vi "Main.vi"() -> ()   [LabVIEW 2019]
doc: "This Continuous Measurement sample project is based on the Queued Message Handler template.\n\nThe Event Handling Loop generates messages based on user interface actions.\n\nThe Message Handling Loop processes messages generated by the Event Handling Loop, or by other messages. There are also Acquisition and Logging message handling loop subVIs, and a chart updating loop."
uses:
  <vilib>/Math Plots/2D Math Plots/2D Compass/2D Compass XCtrl/2D Compass.xctl
  Settings/Settings.ctl
  Acquisition/Hardware Configuration.ctl
  Logging/Logging Configuration.ctl
  controls/UI Data.ctl
  controls/UI Actions.ctl
  controls/UI Info Session.ctl
  Data Analysis/EstimateCluster.ctl
  controls/UI Display.ctl
  controls/Components State.ctl
  controls/State Type.ctl
  controls/Component Type.ctl
  Settings/Session Info.ctl
  controls/UI State.ctl
  support/Message Queue/Enqueue Message (Single).vi
  <vilib>/Utility/xml.llb/Write to XML File(string).vi
  <vilib>/Utility/error.llb/Error Cluster From Error Code.vi
  <vilib>/Utility/xml.llb/Read From XML File(string).vi
  <vilib>/Math Plots/2D Math Plots/2D Plot/2D Plot Datatype/2D Plot Datatype.lvclass
  <vilib>/ErrorRing/Error Ring.xnode
  Acquisition/Acquisition.lvlib
  Settings/Settings.lvlib
  Logging/Logging.lvlib
  support/User Event - Stop/User Event - Stop.lvlib
  support/Message Queue/Message Queue.lvlib
panel:
  out "Etat":string caption="Faux-Taon : Puissance-mètre"
  in  "Note":string
  out "Info sur la session":T1 {"Durée" format="%^<%H:%M:%S>T"}
  in  "Simuler":bool
  in  "Stop":bool
  in  "Start":bool
  in  "Calibrer":bool
  in  "Réinitialiser":bool
  in  "Charger session":bool
  in  "Enregistrer session":bool
  in  "Configuration":T2
  out "Longueur d'onde":dbl
  out "Puissance mesurée":dbl format="%#_3g"
  out "Position instantanée du faisceau vue de face":refnum<class "2D Plot Datatype.lvclass">[](xcontrol) caption="Position instantanée du faisceau"
  out "Graphique des mesures du laser":waveform(dbl)(graph)
  out "Status":string
  in  "Exit":bool
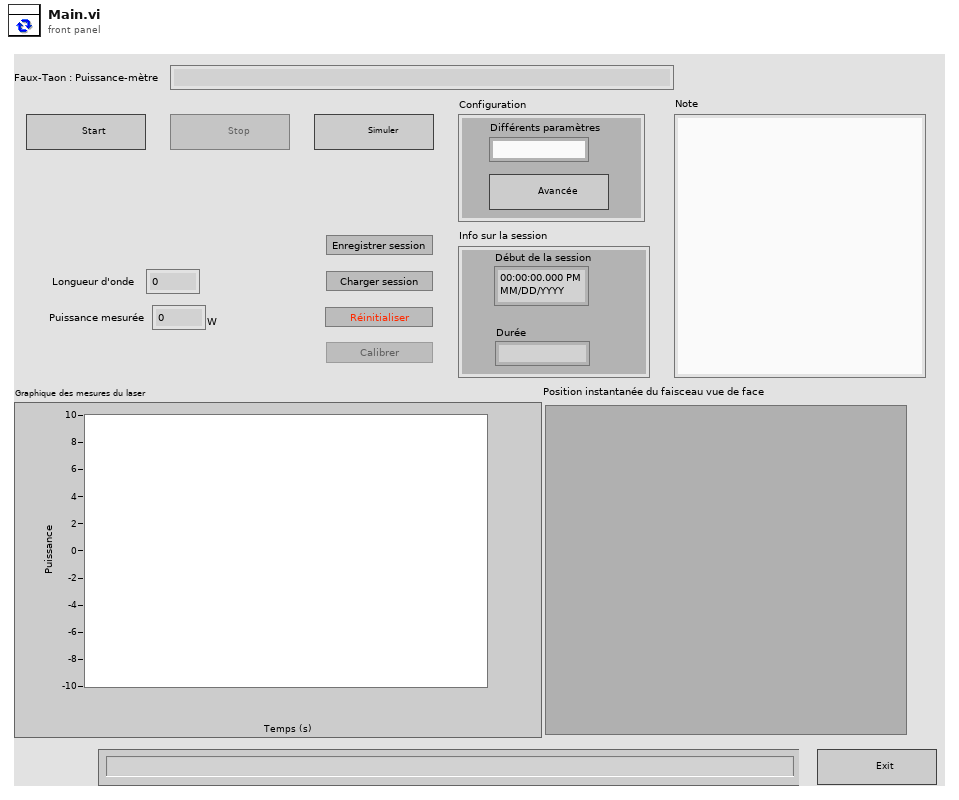
[diagram p1: front panel]
types:
  T1 = cluster{"Début de la session":timestamp, "Durée":timestamp}
  T2 = cluster{"Différents paramètres":string, "Avancée":bool}
  T3 = typedef "Components State.ctl" = cluster{"UI":T4, "Logging":T4, "Acquisition":T4, "Data Analysis":T4, "Estimate Logging":T4, "Data Display":T4}
  T4 = typedef "State Type.ctl" = enum16{"Idle", "Waiting to stop", "Waiting to exit", "Processing", "Exit", "Opened session"}
  T5 = typedef "UI Display.ctl" = cluster{"Graphique des mesures du laser":refnum<vi>, "Position instantanée du faisceau vue de face":refnum<vi>, "Puissance mesurée":refnum<vi>, "Longueur d'onde":refnum<vi>}
  T6 = enum16{"open", "replace", "create", "open or create", "replace or create", "replace or create with confirmation"}
  T7 = typedef "EstimateCluster.ctl" = cluster{"Lambda":dbl, "Puissance":dbl, "Rayon":dbl, "Angle":dbl, "dt":dbl, "t0":timestamp}
  T8 = typedef "UI Data.ctl" = cluster{"Status Ref":refnum<vi>, "Configuration Ref":refnum<vi>, "Action UI":T9, "Info Session":T10}
  T9 = typedef "UI Actions.ctl" = cluster{"Start Ref":refnum<vi>, "Stop Ref":refnum<vi>, "Settings Ref":refnum<vi>, "Exit Ref":refnum<vi>, "Reset Ref":refnum<vi>, "Calibration Ref":refnum<vi>, "Save Ref":refnum<vi>, "Load Ref":refnum<vi>, "Simuler Ref":refnum<vi>}
  T10 = typedef "UI Info Session.ctl" = cluster{"Note Ref":refnum<vi>, "Start Time Ref":refnum<vi>, "Duration Ref":refnum<vi>}
  T11 = typedef "Settings.lvlib/Settings.ctl" = cluster{"Hardware Configuration":T12, "Logging Configuration":T13}
  T12 = typedef "Acquisition.lvlib/Hardware Configuration.ctl" = cluster{"DAQmx Channel":tag, "Max Input":dbl, "Min Input":dbl, "Sample Rate":dbl, "DAQmx Task":refnum<k21>, "Fichier de simulation":path, "Source":enum16{"Simulation", "DAQ"}}
  T13 = typedef "Logging.lvlib/Logging Configuration.ctl" = cluster{"Log File Base Path":path, "DAQ Log TDMS File Reference":refnum<k34>, "Samples to Save":u32, "Trigger - Time":u32, "Trigger - Threshold":dbl, "Trigger - Channel":u32, "Enable Time Trigger":bool, "Enable Threshold Trigger":bool, "Always Log":bool, "Session Name":string, "Estimate Batch Size":i32, "Estimate Filepath":path}
  T14 = typedef "Message Queue.lvlib/All Message Queues.ctl" = cluster{"UI":refnum<queue>, "Components Message Queues":T15}
  T15 = typedef "Message Queue.lvlib/Components Message Queues.ctl" = cluster{"Logging":refnum<queue>, "Acquisition":refnum<queue>, "Data Analysis":refnum<queue>, "Estimate Log":refnum<queue>, "Data Display":refnum<queue>}
  T16 = typedef "Component Type.ctl" = enum16{"UI", "Logging", "Acquisition", "Data Analysis", "Estimate", "Data Display"}
  T17 = typedef "Session Info.ctl" = cluster{"Start time\n":timestamp, "Duration":timestamp, "Note":string}
  T18 = typedef "UI State.ctl" = enum16{"Idle", "Acquiring and Logging", "Waiting for Exit", "Waiting for Exit (Acq Stopped)", "Waiting for Exit (Log Stopped)", "Waiting for Stop", "Waiting for Stop (Acq Stopped)", "Waiting for Stop (Log Stopped)"}
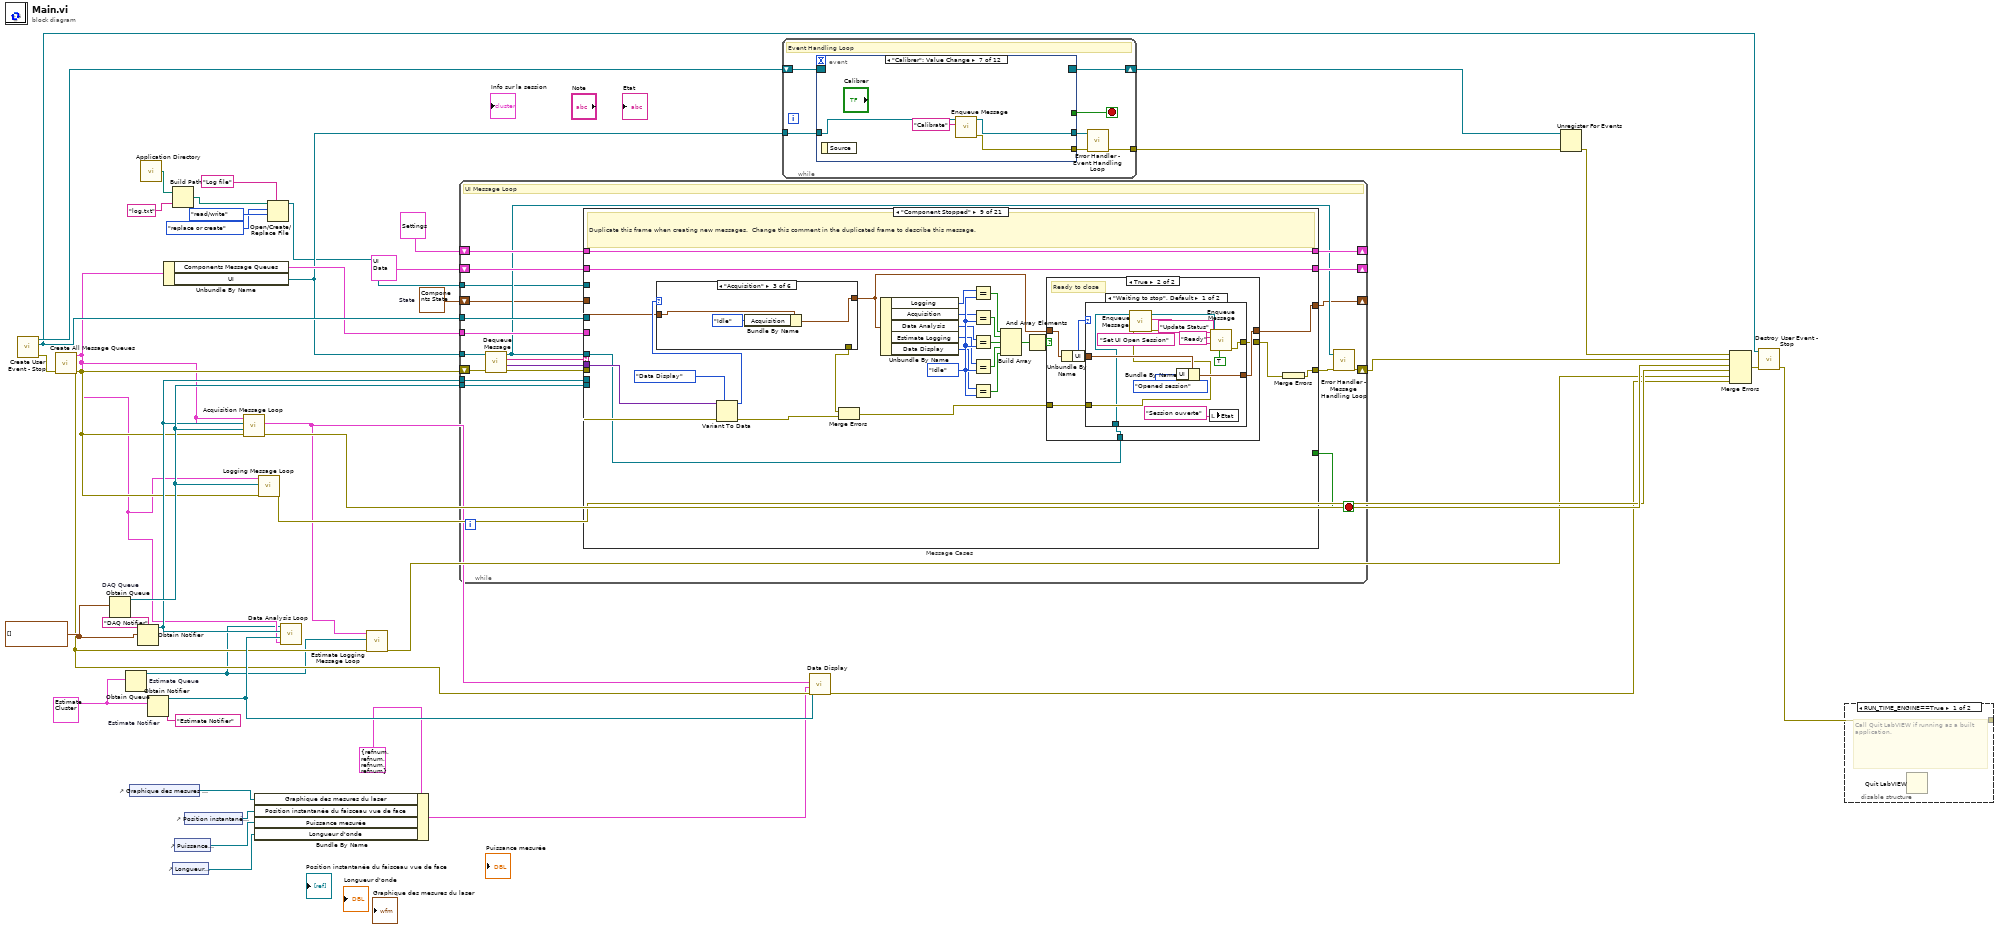
[diagram p0: block diagram]
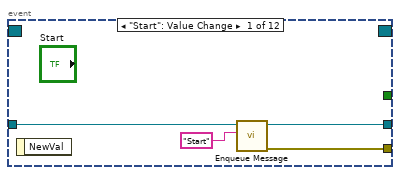
[diagram p3: hidden frame]
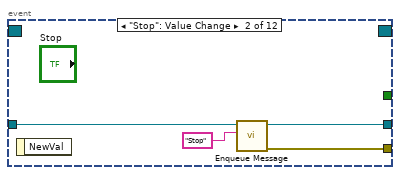
[diagram p4: hidden frame]
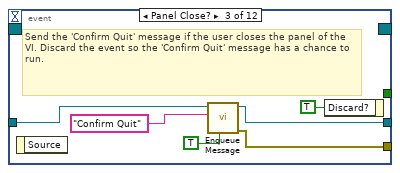
[diagram p5: hidden frame]
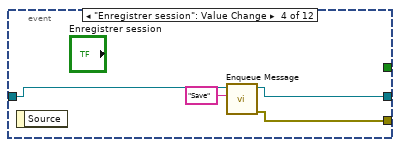
[diagram p6: hidden frame]
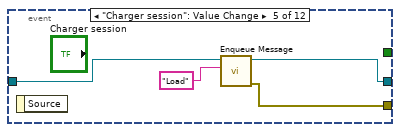
[diagram p7: hidden frame]
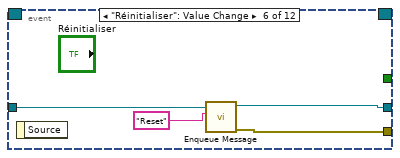
[diagram p8: hidden frame]
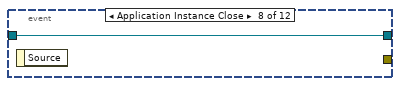
[diagram p9: hidden frame]
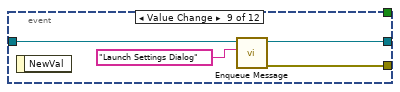
[diagram p10: hidden frame]
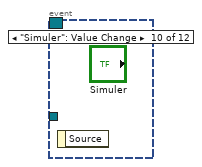
[diagram p11: hidden frame]
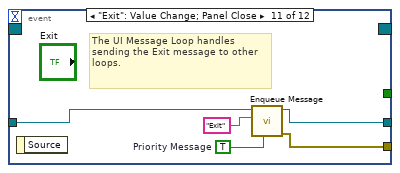
[diagram p12: hidden frame]
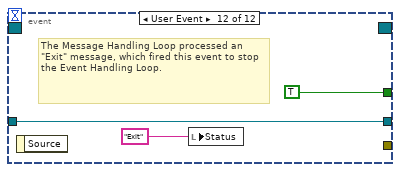
[diagram p13: hidden frame]
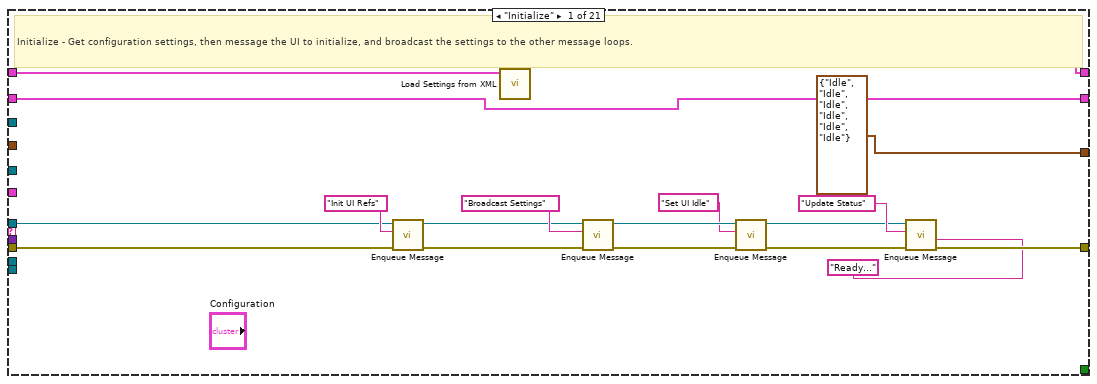
[diagram p14: hidden frame]
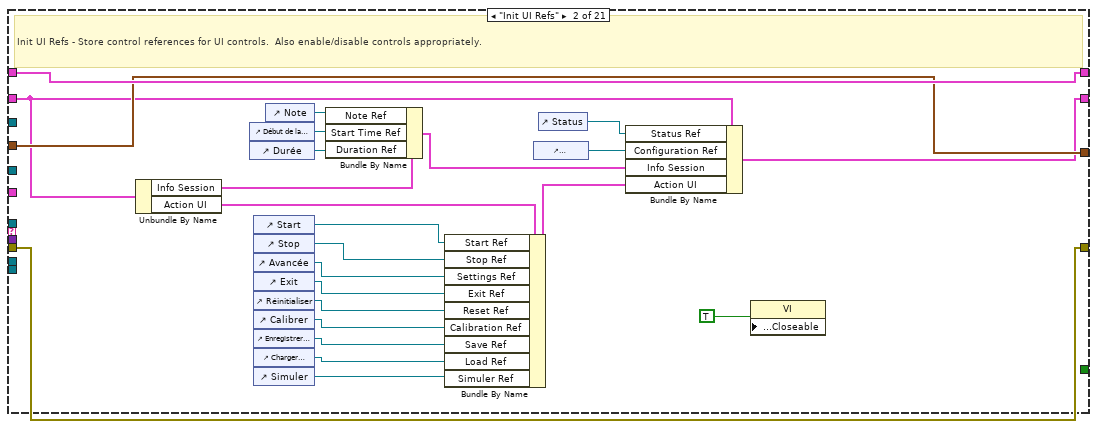
[diagram p15: hidden frame]
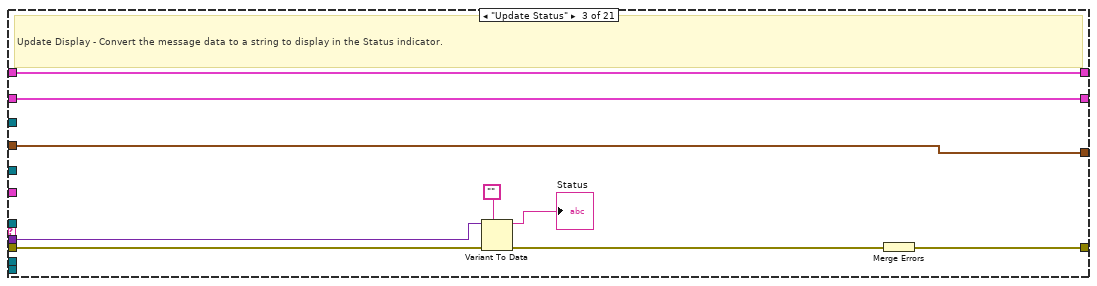
[diagram p16: hidden frame]
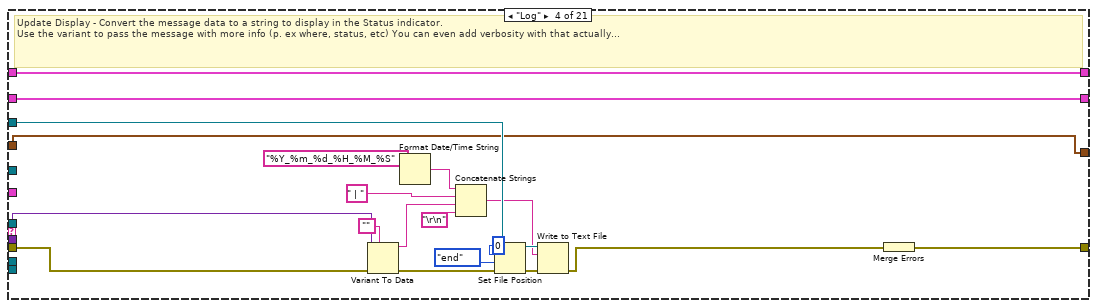
[diagram p17: hidden frame]
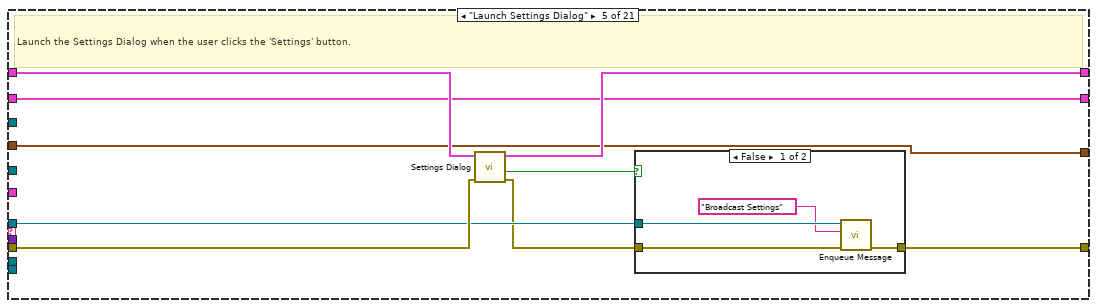
[diagram p18: hidden frame]
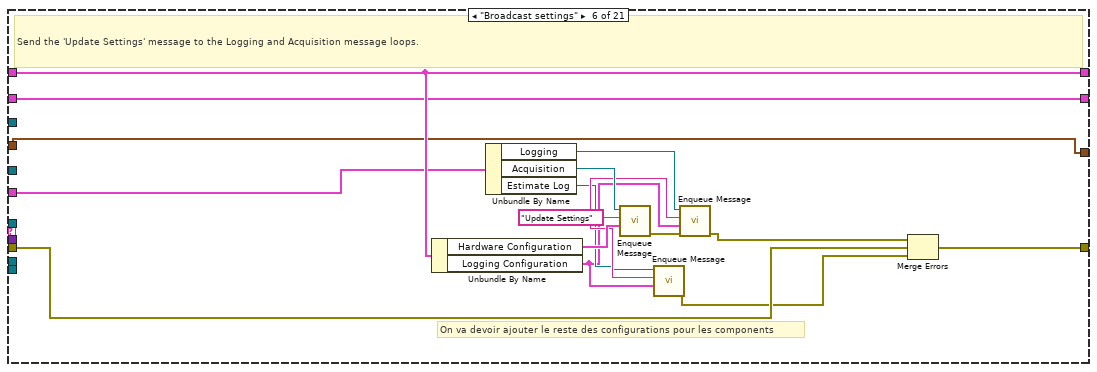
[diagram p20: hidden frame]
diagram:
  w1 = T3 {"UI"=enum."Idle", "Logging"=enum."Idle", "Acquisition"=enum."Idle", "Data Analysis"=enum."Idle", "Estimate Logging"=enum."Idle", "Data Display"=enum."Idle"}  # State
  w22 = T7 {"Lambda"=0.0, "Puissance"=0.0, "Rayon"=0.0, "Angle"=0.0, "dt"=0.0, "t0"=timestamp(0 s since 1904-01-01)} ("Estimate Cluster")
  w24 = waveform(dbl)[] []
  n1 = call "Create User Event - Stop.vi"() -> ("error out"=w35:errorcluster, "User Event - Stop"=w37:refnum<user-event>, "Stop Event Registration Refnum"=w38:refnum<event-registration>)  [unwired: 9 in]
  n2 = call "Create All Message Queues.vi"("error in (no error)"=w35) -> ("error out"=w19:errorcluster, "Message Queues out"=w16:T14)  [unwired: 9 in]
  n3 = Obtain Queue "DAQ Queue"(element data type=w24) -> (queue out=w28:refnum<queue>)  [unwired: 4 in, 2 out]
  n4 = Obtain Queue "Estimate Queue"(element data type=w22) -> (queue out=w2:refnum<queue>)  [unwired: 4 in, 2 out]
  n5 = control-ref of="Graphique des mesures du laser"() -> (w8:refnum<vi>)
  n6 = Obtain Notifier ("DAQ Notifier")(name (unnamed)="DAQ Notifier" ("Logging"), notification data type=w24) -> (notifier out=w20:refnum<notifier>)  [unwired: 2 in, 2 out]
  n7 = call <vilib>:"Application Directory.vi"() -> ("Application Directory"=w12:path)
  n8 = Obtain Notifier "Estimate Notifier"(name (unnamed)="Estimate Notifier", notification data type=w22) -> (notifier out=w21:refnum<notifier>)  [unwired: 2 in, 2 out]
  n9 = Unbundle By Name(w16) -> ("Components Message Queues"=w29:T15, "UI"=w17:refnum<queue>)
  n10 = control-ref of="Longueur d'onde"() -> (w5:refnum<vi>)
  n11 = Build Path(base path=w12, name or relative path="log.txt") -> (appended path=w11:path)
  n12 = control-ref of="Puissance mesurée"() -> (w6:refnum<vi>)
  n13 = control-ref of="Position instantanée du faisceau vue de face"() -> (w7:refnum<vi>)
  n14 = call "Acquisition Message Loop.vi"("error in (no error)"=w19, "Data Queue"=w28, "Data Notifier"=w20, "Message Queues"=w16) -> ("error out"=w36:errorcluster)  [unwired: 7 in]
  n15 = Bundle By Name(cluster=T5 {"Graphique des mesures du laser"=refnum, "Position instantanée du faisceau vue de face"=refnum, "Puissance mesurée"=refnum, "Longueur d'onde"=refnum} ("UI Data Display"), "Graphique des mesures du laser"=w8, "Position instantanée du faisceau vue de face"=w7, "Puissance mesurée"=w6, "Longueur d'onde"=w5) -> (w4:T5)
  n16 = call "Logging Message Loop.vi"("error in (no error)"=w19, "Data Queue"=w28, "Message Queues"=w16) -> ("error out"=w34:errorcluster)  [unwired: 8 in]
  n17 = Open/Create/Replace File(file path (use dialog)=w11, prompt="Log file", operation (0:open)=T6."replace or create", access (0:read/write)=enum16{"read/write", "read-only", "write-only"}."read/write") -> (refnum out=w9:refnum<file>)  [unwired: 2 in, 2 out]
  n18 = call "Data Analysis Loop.vi"("Message Queues"=w16, "Estimate Notifier In"=w21, "DAQ Notifier In"=w20, "Estimate Queue In"=w2) -> ()  [unwired: 6 in, 2 out]
  n19 = call "Estimate Logging Message Loop.vi"("Message Queues"=w16, "Estimate Queue In"=w2, "error in (no error)"=w19) -> ("error out"=w26:errorcluster)  [unwired: 7 in]
  n20 = while {
    tunnel: w17 -> [w55]
    tunnel: w37 -> [w60]
    shift-right: [w46] -> w41
    shift-left: w19 -> [w59]
    shift-right: [w54] -> _
    shift-left: T11 {"Hardware Configuration"={"DAQmx Channel"="", "Max Input"=0.0, "Min Input"=0.0, "Sample Rate"=0.0, "DAQmx Task"="", "Fichier de simulation"=path "", "Source"=enum."Simulation"}, "Logging Configuration"={"Log File Base Path"=path "", "DAQ Log TDMS File Reference"=refnum, "Samples to Save"=0, "Trigger - Time"=0, "Trigger - Threshold"=0.0, "Trigger - Channel"=0, "Enable Time Trigger"=FALSE, "Enable Threshold Trigger"=FALSE, "Always Log"=FALSE, "Session Name"="", "Estimate Batch Size"=0, "Estimate Filepath"=path ""}} ("Settings") -> [w53]
    shift-right: [w51] -> _
    shift-left: T8 {"Status Ref"=refnum, "Configuration Ref"=refnum, "Action UI"={"Start Ref"=refnum, "Stop Ref"=refnum, "Settings Ref"=refnum, "Exit Ref"=refnum, "Reset Ref"=refnum, "Calibration Ref"=refnum, "Save Ref"=refnum, "Load Ref"=refnum, "Simuler Ref"=refnum}, "Info Session"={"Note Ref"=refnum, "Start Time Ref"=refnum, "Duration Ref"=refnum}} ("Measurement UI Controls") -> [w52]
    tunnel: w29 -> [w50]
    tunnel: w20 -> [w49]
    tunnel: w28 -> [w48]
    tunnel: w9 -> [w44]
    shift-right: [w42] -> _
    shift-left: w1 -> [w43]
    stop <- w61 stop-if-true
    # "UI Message Loop"
    n21 = call "Dequeue Message.vi"("error in (no error)"=w59, "Message Queue"=w55) -> ("error out"=w58:errorcluster, "Message Data"=w56:variant, "Message"=w57:string, "dup Message Queue"=w45:refnum<queue>)  [unwired: 6 in]
    n22 = case "Message Cases" shown="\"Component Stopped\"" w57 {
      selector: w57 -> [_ _ _ _ _ _ _ _ _ _ _ _ _ _ _ _ _ _ _ _ w537]
      tunnel: w45 -> [w71 _ _ _ w138 _ w166 w192 w219 w294 _ w390 w403 w439 w453 _ _ _ _ _ _]
      tunnel: w58 -> [w70 w103 w111 w131 w140 w156 w164 w191 w237 w305 w369 w394 w402 w444 w457 w464 w467 w495 w515 w535 _]
      tunnel: [w77 w103 w112 w132 w135 w161 w169 w205 w215 w295 w376 w397 w401 w445 w448 w463 w475 w494 w514 w534 w538] -> w47
      tunnel: [_ _ _ _ _ _ _ _ _ _ _ _ _ TRUE _ _ _ _ _ _ _] -> w61
      tunnel: w56 -> [_ _ w110 w130 _ _ _ _ w238 _ _ _ _ _ w456 _ _ _ _ _ _]
      tunnel: w60 -> [_ _ _ _ _ _ _ _ _ _ _ _ _ w443 _ _ _ _ _ _ _]
      tunnel: [w78 w102 w107 w128 w137 w159 w177 w210 w241 w298 w374 w396 w405 w442 w459 w462 w474 w493 w513 w533 w540] -> w54
      tunnel: w53 -> [w79 w102 w107 w128 w141 w159 w177 w210 w241 w299 w374 w396 w405 w442 w459 w462 w474 w493 w513 w533 w540]
      tunnel: w52 -> [w73 w98 w106 w127 w134 w155 w185 w195 w240 w300 w358 w387 w404 w440 w458 w461 w473 w477 w498 w521 w539]
      tunnel: [w73 w99 w106 w127 w134 w155 w185 w195 w240 w300 w358 w387 w404 w440 w458 w461 w473 w477 w498 w521 w539] -> w51
      tunnel: w50 -> [_ _ _ _ _ w154 w184 w204 _ w297 _ w395 _ w432 _ _ w471 _ _ _ _]
      tunnel: w49 -> [_ _ _ _ _ _ _ _ _ _ _ _ _ w438 _ _ _ _ _ _ _]
      tunnel: w48 -> [_ _ _ _ _ _ _ _ _ _ _ _ _ w434 _ _ _ _ _ _ _]
      tunnel: w44 -> [_ _ _ w123 _ _ _ _ _ _ _ _ _ _ _ _ _ _ _ _ _]
      tunnel: w43 -> [_ w100 w104 w113 w133 w147 _ w201 w234 w304 w375 w392 w399 w430 w447 w460 w472 w492 w512 w532 w536]
      tunnel: [T3 {"UI"=enum."Idle", "Logging"=enum."Idle", "Acquisition"=enum."Idle", "Data Analysis"=enum."Idle", "Estimate Logging"=enum."Idle", "Data Display"=enum."Idle"} ("State") w100 w104 w113 w133 w147 T3 {"UI"=enum."Processing", "Logging"=enum."Processing", "Acquisition"=enum."Processing", "Data Analysis"=enum."Processing", "Estimate Logging"=enum."Processing", "Data Display"=enum."Processing"} ("State") w202 w220 w304 w375 w392 w398 w430 w447 w460 w472 w492 w512 w532 w536] -> w42
      frame "Initialize" {
        # "Initialize - Get configuration settings, then message the UI to initialize, and broadcast the settings to the other message loops."
        n23 = call-poly "Enqueue Message.vi"("error in (no error)"=w70, "Message"="Init UI Refs", "Message Queue"=w71) -> ("error out"=w68:errorcluster, "dup Message Queue"=w69:refnum<queue>)  [unwired: 7 in]
        n24 = call "Load Settings from XML.vi"("Settings in"=w79) -> ("Settings out"=w78:T11)  [unwired: 9 in, 1 out]
        n25 = call-poly "Enqueue Message.vi"("error in (no error)"=w68, "Message"="Broadcast Settings", "Message Queue"=w69) -> ("error out"=w64:errorcluster, "dup Message Queue"=w66:refnum<queue>)  [unwired: 7 in]
        n26 = call-poly "Enqueue Message.vi"("error in (no error)"=w64, "Message"="Set UI Idle", "Message Queue"=w66) -> ("error out"=w63:errorcluster, "dup Message Queue"=w65:refnum<queue>)  [unwired: 7 in]
        n27 = call-poly "Enqueue Message.vi"("error in (no error)"=w63, "Message Data"="Ready..." ("Ready..."), "Message"="Update Status", "Message Queue"=w65) -> ("error out"=w77:errorcluster)  [unwired: 6 in, 1 out]
      }
      frame "Init UI Refs" {
        # "Init UI Refs - Store control references for UI controls.  Also enable/disable controls appropriately."
        n28 = Unbundle By Name(w98) -> ("Info Session"=w97:T10, "Action UI"=w96:T9)
        n29 = control-ref of="Début de la session"() -> (w94:refnum<vi>)
        n30 = control-ref of="Durée"() -> (w80:refnum<vi>)
        n31 = control-ref of="Start"() -> (w85:refnum<vi>)
        n32 = control-ref of="Stop"() -> (w84:refnum<vi>)
        n33 = control-ref of="Avancée"() -> (w86:refnum<vi>)
        n34 = control-ref of="Exit"() -> (w87:refnum<vi>)
        n35 = control-ref of="Réinitialiser"() -> (w83:refnum<vi>)
        n36 = control-ref of="Calibrer"() -> (w88:refnum<vi>)
        n37 = control-ref of="Enregistrer session"() -> (w82:refnum<vi>)
        n38 = control-ref of="Charger session"() -> (w89:refnum<vi>)
        n39 = control-ref of="Simuler"() -> (w81:refnum<vi>)
        n40 = control-ref of="Note"() -> (w95:refnum<vi>)
        n41 = Bundle By Name(cluster=w97, "Note Ref"=w95, "Start Time Ref"=w94, "Duration Ref"=w80) -> (w93:T10)
        n42 = Bundle By Name(cluster=w96, "Start Ref"=w85, "Stop Ref"=w84, "Settings Ref"=w86, "Exit Ref"=w87, "Reset Ref"=w83, "Calibration Ref"=w88, "Save Ref"=w82, "Load Ref"=w89, "Simuler Ref"=w81) -> (w92:T9)
        n43 = control-ref of="Configuration"() -> (w91:refnum<vi>)
        n44 = control-ref of="Status"() -> (w90:refnum<vi>)
        n45 = Bundle By Name(cluster=w98, "Status Ref"=w90, "Configuration Ref"=w91, "Info Session"=w93, "Action UI"=w92) -> (w99:T8)
        n46 = property class="VI"("Front Panel.Closeable"=TRUE ("Front Panel Window:Closeable")) -> ()  [unwired: 2 in, 2 out]
      }
      frame "Update Status" {
        # "Update Display - Convert the message data to a string to display in the Status indicator."
        n47 = Variant To Data(error in=w111, type="", Variant=w110) -> (data=→"Status":string, error out=w108:errorcluster)
        n48 = Merge Errors(w108) -> (w112:errorcluster)
      }
      frame "Log" {
        # "Update Display - Convert the message data to a string to display in the Status indicator.\nUse the variant to pass the message with more info (p. ex where, status, etc) You can even add verbosity with that actually..."
        n49 = Variant To Data(error in=w131, type="", Variant=w130) -> (data=w122:string, error out=w119:errorcluster)
        n50 = Format Date/Time String(time format string (%c)="%Y_%m_%d_%H_%M_%S") -> (date/time string=w115:string)  [unwired: 2 in]
        n51 = Concatenate Strings(w115, " | " ("string"), w122, "\r\n") -> (w120:string)
        n52 = Set File Position(offset (in bytes) (0)=i64 0, refnum=w123, from (0:start)=enum16{"start", "end", "current"}."end", error in=w119) -> (refnum out=w126:refnum<file>, error out=w118:errorcluster)
        n53 = Write to Text File(file (use dialog)=w126, text=w120, error in=w118) -> (error out=w117:errorcluster)  [unwired: 1 in, 2 out]
        n54 = Merge Errors(w117) -> (w132:errorcluster)
      }
      frame "Launch Settings Dialog" {
        # "Launch the Settings Dialog when the user clicks the 'Settings' button."
        n55 = call "Settings Dialog.vi"("error in (no error)"=w140, "Settings in"=w141) -> ("error out"=w136:errorcluster, "Cancelled?"=w139:bool, "Settings out"=w137:T11)  [unwired: 6 in, 1 out]
        n56 = case shown="False" w139 {
          tunnel: w138 -> [w145 _]
          tunnel: w136 -> [w144 w146]
          tunnel: [w143 w146] -> w135
          frame False {
            n57 = call-poly "Enqueue Message.vi"("error in (no error)"=w144, "Message"="Broadcast Settings", "Message Queue"=w145) -> ("error out"=w143:errorcluster)  [unwired: 7 in, 1 out]
          }
          frame True {
          }
        }
      }
      frame "Broadcast settings" {
        w151 = "Update Settings" ("Message")
        # "On va devoir ajouter le reste des configurations pour les components"
        # "Send the 'Update Settings' message to the Logging and Acquisition message loops."
        n58 = Unbundle By Name(w159) -> ("Hardware Configuration"=w158:T12, "Logging Configuration"=w149:T13)
        n59 = Unbundle By Name(w154) -> ("Logging"=w152:refnum<queue>, "Acquisition"=w153:refnum<queue>, "Estimate Log"=w150:refnum<queue>)
        n60 = call-poly "Enqueue Message.vi"("Message Data"=w158, "Message"=w151, "Message Queue"=w153) -> ("error out"=w160:errorcluster)  [unwired: 7 in, 1 out]
        n61 = call-poly "Enqueue Message.vi"("Message Data"=w149, "Message"=w151, "Message Queue"=w150) -> ("error out"=w148:errorcluster)  [unwired: 7 in, 1 out]
        n62 = call-poly "Enqueue Message.vi"("error in (no error)"=w160, "Message Data"=w149, "Message"=w151, "Message Queue"=w152) -> ("error out"=w157:errorcluster)  [unwired: 6 in, 1 out]
        n63 = Merge Errors(w157, w156, w148) -> (w161:errorcluster)
      }
      frame "Start" {
        # "Start - Enable/Disable buttons appropriately for an acquisition that has started, and update status display. Also log the config.\n\nMight want to set all the filenames right away"
        n64 = call-poly "Enqueue Message.vi"("error in (no error)"=w164, "Message"="Set UI Running", "Message Queue"=w166) -> ("error out"=w163:errorcluster, "dup Message Queue"=w165:refnum<queue>)  [unwired: 7 in]
        n65 = Unbundle By Name(w177) -> ("Logging Configuration.Log File Base Path"=w181:path, "Logging Configuration.Session Name"=w180:string)
        n66 = call-poly "Enqueue Message.vi"("error in (no error)"=w163, "Message Data"="Waiting for trigger" ("Waiting for trigger"), "Message"="Update Status", "Message Queue"=w165) -> ("error out"=w182:errorcluster)  [unwired: 6 in, 1 out]
        n67 = Unbundle By Name(w185) -> ("Info Session.Start Time Ref"=w172:refnum<vi>)
        n68 = Build Path(base path=w181, name or relative path=w180) -> (appended path=w179:path)
        n69 = Get Date/Time In Seconds() -> (seconds since 1Jan1904=w171:timestamp)
        n70 = call "Enqueue Message (All Components).vi"("error in (no error)"=w182, "Message"="Start", "Components Message Queues"=w184) -> ("error out"=w174:errorcluster)  [unwired: 8 in]
        n71 = Build Path(base path=w179, name or relative path="Settings.xml") -> (appended path=w175:path)
        n72 = Flatten To XML(anything=w177) -> (xml string=w176:string)
        n73 = property class="AbsTime (strict)"(reference=w172, "Value"=w171) -> (error out=w168:errorcluster)  [unwired: 1 in, 1 out]
        n74 = call-poly <vilib>:"Write to XML File.vi"("error in (no error)"=w174, "XML Input"=w176, "XML File Path"=w175) -> ("error out"=w170:errorcluster)  [unwired: 6 in, 2 out]
        n75 = Merge Errors(w168, w170) -> (w169:errorcluster)
        n76 = local write "Etat"("Acquisition en cours" ("Etat")) -> ()
      }
      frame "Stop" {
        # "Stop - Enable/Disable buttons appropriately for an acquisition that has stopped, and update status display."
        n77 = Unbundle By Name(w195) -> ("Action UI.Stop Ref"=w189:refnum<vi>, "Info Session.Start Time Ref"=w197:refnum<vi>, "Info Session.Duration Ref"=w198:refnum<vi>)
        n78 = Unbundle By Name(w201) -> ("UI"=w203:T4)
        n79 = property class="AbsTime (strict)"(reference=w197) -> ("Value"=w196:timestamp)  [unwired: 1 in, 2 out]
        n80 = Get Date/Time In Seconds() -> (seconds since 1Jan1904=w199:timestamp)
        n81 = Subtract(x=w199, y=w196) -> (x-y=w194:dbl)
        n82 = Build Array(w189) -> (w188:refnum<vi>[])
        n83 = To Time Stamp(1:w194) -> (0:w193:timestamp)
        n84 = call "Set Enable State on Multiple Controls.vi"("Enable?"=FALSE, "Controls"=w188) -> ()  [unwired: 10 in]
        n85 = property class="AbsTime (strict)"(reference=w198, "Value"=w193) -> ()  [unwired: 1 in, 2 out]
        n86 = call-poly "Enqueue Message.vi"("error in (no error)"=w191, "Message Data"="Arrêt en cours" ("Ready..."), "Message"="Update Status", "Message Queue"=w192) -> ("error out"=w207:errorcluster)  [unwired: 6 in, 1 out]
        n87 = call-poly "Enqueue Message.vi"("error in (no error)"=w207, "Message"="Stop", "Components Message Queues"=w204) -> ("error out"=w205:errorcluster)  [unwired: 8 in]
        n88 = case shown="Default" w203 {
          tunnel: [T3 {"UI"=enum."Waiting to stop", "Logging"=enum."Waiting to stop", "Acquisition"=enum."Waiting to stop", "Data Analysis"=enum."Waiting to stop", "Estimate Logging"=enum."Waiting to stop", "Data Display"=enum."Waiting to stop"} ("State") w212 w213] -> w202
          tunnel: w201 -> [_ w212 w213]
          frame Default {
          }
          frame "Waiting to exit" {
          }
          frame "Waiting to stop" {
          }
        }
        n89 = local write "Etat"("Acquisition en cours d'arrêt" ("Etat")) -> ()
      }
      frame "Component Stopped" {
        w232 = State_Type."Idle" ("y")
        # "Duplicate this frame when creating new messages.  Change this comment in the duplicated frame to describe this message."
        n90 = Variant To Data(error in=w237, type=Component_Type."Data Display" ("Component Type"), Variant=w238) -> (data=w235:T16, error out=w236:errorcluster)
        n91 = case shown="\"Acquisition\"" w235 {
          selector: w235 -> [w270 _ _ _ _ _]
          tunnel: w234 -> [w268 w280 w282 w285 w287 w290]
          tunnel: [w269 _ _ _ _ _] -> w218
          tunnel: [w268 w278 w281 w284 w288 w291] -> w217
          frame "UI", Default {
            n92 = xnode "Error Ring"("parameter 0"=w270) -> ("error out"=w269:errorcluster)
          }
          frame "Logging" {
            n93 = Bundle By Name(cluster=w280, "Logging"=State_Type."Idle") -> (w278:T3)
          }
          frame "Acquisition" {
            n94 = Bundle By Name(cluster=w282, "Acquisition"=State_Type."Idle" ("Logging")) -> (w281:T3)
          }
          frame "Data Analysis" {
            n95 = Bundle By Name(cluster=w285, "Data Analysis"=State_Type."Idle" ("Logging")) -> (w284:T3)
          }
          frame "Estimate" {
            n96 = Bundle By Name(cluster=w287, "Estimate Logging"=State_Type."Idle" ("Logging")) -> (w288:T3)
          }
          frame "Data Display" {
            n97 = Bundle By Name(cluster=w290, "Data Display"=State_Type."Idle" ("Logging")) -> (w291:T3)
          }
        }
        n98 = Merge Errors(w218, w236) -> (w216:errorcluster)
        n99 = Unbundle By Name(w217) -> ("Logging"=w233:T4, "Acquisition"=w231:T4, "Data Analysis"=w230:T4, "Estimate Logging"=w229:T4, "Data Display"=w228:T4)
        n100 = Equal?(x=w233, y=w232) -> (x = y?=w227:bool)
        n101 = Equal?(x=w231, y=w232) -> (x = y?=w226:bool)
        n102 = Equal?(x=w230, y=w232) -> (x = y?=w225:bool)
        n103 = Equal?(x=w229, y=w232) -> (x = y?=w224:bool)
        n104 = Equal?(x=w228, y=w232) -> (x = y?=w223:bool)
        n105 = Build Array(w227, w226, w225, w224, w223) -> (w222:bool[])
        n106 = And Array Elements(Boolean array=w222) -> (logical AND=w221:bool)
        n107 = case shown="True" w221 {
          tunnel: w217 -> [w243 w247]
          tunnel: [w243 w249] -> w220
          tunnel: w219 -> [_ w246]
          tunnel: w216 -> [w242 w245]
          tunnel: [w242 w244] -> w214
          frame False {
          }
          frame True {
            # "Ready to close"
            n108 = Unbundle By Name(w247) -> ("UI"=w248:T4)
            n109 = case shown="\"Waiting to stop\", Default" w248 {
              tunnel: [w262 w264] -> w249
              tunnel: w247 -> [w260 w264]
              tunnel: w246 -> [w250 w266]
              tunnel: w245 -> [w254 _]
              tunnel: [w252 w263] -> w244
              frame "Waiting to stop", Default {
                n110 = call-poly "Enqueue Message.vi"("error in (no error)"=w254, "Message"="Set UI Open Session", "Message Queue"=w250) -> ("error out"=w253:errorcluster, "dup Message Queue"=w251:refnum<queue>)  [unwired: 7 in]
                n111 = Bundle By Name(cluster=w260, "UI"=State_Type."Opened session") -> (w262:T3)
                n112 = local write "Etat"("Session ouverte" ("Etat")) -> ()
                n113 = call-poly "Enqueue Message.vi"("Priority Message? (F)"=TRUE, "error in (no error)"=w253, "Message Data"="Ready" ("Message"), "Message"="Update Status", "Message Queue"=w251) -> ("error out"=w252:errorcluster)  [unwired: 5 in, 1 out]
              }
              frame "Waiting to exit" {
                n114 = call-poly "Enqueue Message.vi"("Priority Message? (F)"=TRUE, "Message"="Exit", "Message Queue"=w266) -> ("error out"=w263:errorcluster)  [unwired: 7 in, 1 out]
              }
            }
          }
        }
        n115 = Merge Errors(w214) -> (w215:errorcluster)
      }
      frame "Load" {
        # "Info should hold all the info regarding the session as well as filename. Then we validate existence before sending the filepathé"
        # "Charger toutes les infos, gérer les états de l'UI etc\nConfig, Info et passe le message aux components"
        n116 = call <vilib>:"Application Directory.vi"() -> ("Application Directory"=w303:path)
        n117 = call "File Dialog"("start path"=w303, "prompt"="Veuillez choisir le dossier contenant la session à ouvrir.", "pattern (all files)"="*.dir") -> ("selected path"=w296:path, "cancelled"=w293:bool)  [unwired: 9 in, 2 out]
        n118 = case shown="False" w293 {
          tunnel: w305 -> [w338 w342]
          tunnel: w300 -> [w332 _]
          tunnel: w299 -> [w320 w344]
          tunnel: [w319 w344] -> w298
          tunnel: w297 -> [w312 _]
          tunnel: w296 -> [w310 _]
          tunnel: [w308 w341] -> w295
          tunnel: w294 -> [w307 w343]
          frame False {
            # "Actually, not all config should be loaded. p. ex. temp folder. \nJust those selected by the user"
            n119 = Build Path(base path=w310, name or relative path="Settings.xml") -> (appended path=w324:path)
            n120 = Build Path(base path=w310, name or relative path="Info.xml") -> (appended path=w335:path)
            n121 = call-poly <vilib>:"Read From XML File.vi"("XML File Path"=w324) -> ("error out"=w322:errorcluster, "XML Elements"=w323:string)  [unwired: 8 in, 1 out]
            n122 = call-poly <vilib>:"Read From XML File.vi"("XML File Path"=w335) -> ("error out"=w321:errorcluster, "XML Elements"=w334:string)  [unwired: 8 in, 1 out]
            n123 = Unbundle By Name(w332) -> ("Info Session.Note Ref"=w331:refnum<vi>, "Info Session.Start Time Ref"=w330:refnum<vi>, "Info Session.Duration Ref"=w329:refnum<vi>)
            n124 = Unflatten From XML(xml string=w334, type=T17 {"Start time\n"=timestamp(0 s since 1904-01-01), "Duration"=timestamp(0 s since 1904-01-01), "Note"=""} ("Session Info"), error in (no error)=w321) -> (value=w328:T17, error out=w317:errorcluster)
            n125 = Unflatten From XML(xml string=w323, type=w320, error in (no error)=w322) -> (value=w319:T11, error out=w318:errorcluster)
            n126 = Unbundle By Name(w328) -> ("Start time"=w325:timestamp, "Duration"=w326:timestamp, "Note"=w327:string)
            n127 = property class="Str"(reference=w331, error in=w317, "Value"=w327) -> (error out=w314:errorcluster)  [unwired: 1 out]
            n128 = property class="AbsTime (strict)"(reference=w330, error in=w317, "Value"=w325) -> (error out=w315:errorcluster)  [unwired: 1 out]
            n129 = property class="AbsTime (strict)"(reference=w329, error in=w317, "Value"=w326) -> (error out=w316:errorcluster)  [unwired: 1 out]
            n130 = Merge Errors(w314, w315, w316, w338, w318) -> (w313:errorcluster)
            n131 = call "Enqueue Message (All Components).vi"("error in (no error)"=w313, "Message Data"=w310, "Message"="Load", "Components Message Queues"=w312) -> ("error out"=w309:errorcluster)  [unwired: 7 in]
            n132 = call-poly "Enqueue Message.vi"("error in (no error)"=w309, "Message"="Set UI Open Session", "Message Queue"=w307) -> ("error out"=w308:errorcluster)  [unwired: 7 in, 1 out]
          }
          frame True {
            n133 = call-poly "Enqueue Message.vi"("error in (no error)"=w342, "Message Data"="Le chargement de la session a été annulé." ("Message"), "Message"="Update Status", "Message Queue"=w343) -> ("error out"=w341:errorcluster)  [unwired: 6 in, 1 out]
          }
        }
      }
      frame "Save" {
        # "On ne peut pas sauvegarder deux fois la même session; les fichiers ont été déplacés. Vérifier ce qui se passe pour Move et Copy though\nAnswer. It crashes"
        # "Cauntion. All component must be idle ideally. If it's in the process of stopping, you might be in a problem. Might be better not to ask for folder\n- Move unlocking the button to Component closed when it's confirmed.\n- Add status (Open session) to clarify process"
        n134 = Unbundle By Name(w358) -> ("Action UI.Save Ref"=w361:refnum<vi>)
        n135 = Unbundle By Name(w358) -> ("Info Session.Start Time Ref"=w357:refnum<vi>, "Info Session.Duration Ref"=w356:refnum<vi>, "Info Session.Note Ref"=w355:refnum<vi>)
        n136 = Unbundle By Name(w374) -> ("Logging Configuration.Log File Base Path"=w373:path, "Logging Configuration.Session Name"=w372:string)
        n137 = Build Array(w361) -> (w360:refnum<vi>[])
        n138 = call "Set Enable State on Multiple Controls.vi"("Enable?"=FALSE, "Controls"=w360) -> ()  [unwired: 10 in]
        n139 = property class="AbsTime (strict)"(reference=w357) -> ("Value"=w354:timestamp)  [unwired: 1 in, 2 out]
        n140 = property class="AbsTime (strict)"(reference=w356) -> ("Value"=w353:timestamp)  [unwired: 1 in, 2 out]
        n141 = property class="Str"(reference=w355) -> ("Value"=w352:string)  [unwired: 1 in, 2 out]
        n142 = Build Path(base path=w373, name or relative path=w372) -> (appended path=w371:path)
        n143 = Move(source path=w371, error in=w369, 7:"Veuillez choisir le dossier où enregistrer la session en cours." ("prompt (Create Folder)")) -> (error out=w365:errorcluster, 3:w349:path)  [unwired: 2 in, 1 out]
        n144 = Bundle By Name(cluster=T17 {"Start time\n"=timestamp(0 s since 1904-01-01), "Duration"=timestamp(0 s since 1904-01-01), "Note"=""} ("Session Info"), "Start time"=w354, "Duration"=w353, "Note"=w352) -> (w350:T17)
        n145 = Flatten To XML(anything=w350) -> (xml string=w346:string)
        n146 = call <vilib>:"Application Directory.vi"() -> ("Application Directory"=w368:path)
        n147 = Build Path(base path=w368, name or relative path="log.txt") -> (appended path=w367:path)
        n148 = Build Path(base path=w349, name or relative path="log.txt") -> (appended path=w363:path)
        n149 = Build Path(base path=w349, name or relative path="Info.xml") -> (appended path=w347:path)
        n150 = Copy(8:w365, 10:w363, 11:w367) -> (0:w359:errorcluster)  [unwired: 2 in, 2 out]
        n151 = call-poly <vilib>:"Write to XML File.vi"("XML Input"=w346, "XML File Path"=w347) -> ("error out"=w345:errorcluster)  [unwired: 7 in, 2 out]
        n152 = Merge Errors(w359, w345) -> (w376:errorcluster)
      }
      frame "Reset" {
        # "Remet tous les composants à 0"
        n153 = call-poly "Enqueue Message.vi"("error in (no error)"=w394, "Message"="Reset", "Components Message Queues"=w395) -> ("error out"=w383:errorcluster)  [unwired: 8 in]
        n154 = Unbundle By Name(w387) -> ("Info Session.Note Ref"=w386:refnum<vi>, "Info Session.Start Time Ref"=w385:refnum<vi>, "Info Session.Duration Ref"=w384:refnum<vi>)
        n155 = property class="Str"(reference=w386, error in=w383, "Value"="") -> (error out=w382:errorcluster)  [unwired: 1 out]
        n156 = property class="AbsTime (strict)"(reference=w385, error in=w382, "Value"=timestamp(0 s since 1904-01-01)) -> (error out=w381:errorcluster)  [unwired: 1 out]
        n157 = property class="AbsTime (strict)"(reference=w384, error in=w381, "Value"=timestamp(0 s since 1904-01-01)) -> (error out=w380:errorcluster)  [unwired: 1 out]
        n158 = call-poly "Enqueue Message.vi"("error in (no error)"=w380, "Message"="Set UI Idle", "Message Queue"=w390) -> ("error out"=w389:errorcluster)  [unwired: 7 in, 1 out]
        n159 = local write "Etat"("Prêt" ("Etat")) -> ()
        n160 = Merge Errors(w389) -> (w397:errorcluster)
      }
      frame "Confirm Quit" {
        # "Confirm Quit - Message that can confirm whether or not the user wants to exit the application. -> Panel close?"
        n161 = Unbundle By Name(w399) -> ("UI"=w400:T4)
        n162 = case shown="\"Processing\"" w400 {
          tunnel: w403 -> [w411 w417]
          tunnel: w402 -> [w410 w415]
          tunnel: [w407 w414] -> w401
          tunnel: w399 -> [w406 w413]
          tunnel: [w406 w412] -> w398
          frame Default {
            # "If 'Confirm Quit' comes in while the system is idle, there is no need for a confirmation message."
            n163 = call-poly "Enqueue Message.vi"("Priority Message? (F)"=TRUE, "error in (no error)"=w410, "Message"="Exit", "Message Queue"=w411) -> ("error out"=w407:errorcluster)  [unwired: 6 in, 1 out]
          }
          frame "Processing" {
            n164 = Two Button Dialog(message="Are you sure you want to quit while the acquisition is running?" ("Confirm Quit Message"), 1:"No" ("No"), 2:"Yes" ("Yes")) -> (T button?=w416:bool)
            n165 = case shown="False" w416 {
              tunnel: w417 -> [_ w429]
              tunnel: w415 -> [w422 w428]
              tunnel: [w422 w427] -> w414
              tunnel: w413 -> [w421 w425]
              tunnel: [w421 w424] -> w412
              frame False {
                # "User did not want to quit."
              }
              frame True {
                n166 = call-poly "Enqueue Message.vi"("error in (no error)"=w428, "Message"="Stop", "Message Queue"=w429) -> ("error out"=w427:errorcluster)  [unwired: 7 in, 1 out]
                n167 = Bundle By Name(cluster=w425, "UI"=State_Type."Waiting to exit") -> (w424:T3)
              }
            }
          }
        }
      }
      frame "Exit" {
        (unwired) UI_State."Idle" ("UI State")
        # "Don't check the error outs. The queues may have already been released."
        # "Close references owned by the Main VI."
        # "Stop the VI"
        # "Exit - Fire the User Event to stop the Event Handling Loop.  Also send Exit messages to the Acquisition and Logging loops."
        n168 = Release Queue(queue=w439, error in (no error)=w444) -> (error out=w437:errorcluster)  [unwired: 1 in, 2 out]
        n169 = call "Fire User Event - Stop.vi"("User Event - Stop"=w443) -> ("error out"=w431:errorcluster)  [unwired: 10 in]
        n170 = Release Notifier(notifier=w438, error in (no error)=w437) -> (error out=w436:errorcluster)  [unwired: 1 in, 2 out]
        n171 = Release Queue(queue=w434, error in (no error)=w436) -> (error out=w435:errorcluster)  [unwired: 1 in, 2 out]
        n172 = call-poly "Enqueue Message.vi"("Priority Message? (F)"=TRUE, "Message"="Exit", "Components Message Queues"=w432) -> ()  [unwired: 8 in, 1 out]
        n173 = Merge Errors(w431, w435) -> (w445:errorcluster)
      }
      frame "Error" {
        # "Error - Check the error message data and respond accordingly. This message is sent by the \"Error Handler\" VIs at the end of each loop in this application."
        n174 = Variant To Data(error in=w457, type=errorcluster {"status"=FALSE, "code"=0, "source"=""} ("error out"), Variant=w456) -> (data=w454:errorcluster, error out=w450:errorcluster)
        n175 = call <vilib>:"Simple Error Handler.vi"("error in (no error)"=w454) -> ()  [unwired: 4 in, 5 out]
        n176 = call-poly "Enqueue Message.vi"("Priority Message? (F)"=TRUE, "Message"="Exit", "Message Queue"=w453) -> ("error out"=w449:errorcluster)  [unwired: 7 in, 1 out]
        n177 = Merge Errors(w449, w450) -> (w448:errorcluster)
      }
      frame "---Copy This Frame---" {
        # "Duplicate this frame when creating new messages.  Change this comment in the duplicated frame to describe this message."
        n178 = Merge Errors(w464) -> (w463:errorcluster)
      }
      frame "Calibrate" {
        w468 = "Calibrate" ("Message")
        # "Ask acquisition for one value. Send Data Analysis Calibrate instruction"
        n179 = Unbundle By Name(w471) -> ("Data Analysis"=w469:refnum<queue>, "Acquisition"=w470:refnum<queue>)
        n180 = call-poly "Enqueue Message.vi"("error in (no error)"=w467, "Message"=w468, "Message Queue"=w470) -> ("error out"=w466:errorcluster)  [unwired: 7 in, 1 out]
        n181 = call-poly "Enqueue Message.vi"("error in (no error)"=w466, "Message"=w468, "Message Queue"=w469) -> ("error out"=w465:errorcluster)  [unwired: 7 in, 1 out]
        n182 = Merge Errors(w465) -> (w475:errorcluster)
      }
      frame "Set UI Idle" {
        # "Duplicate this frame when creating new messages.  Change this comment in the duplicated frame to describe this message."
        n183 = Unbundle By Name(w477) -> ("Status Ref"=w491:refnum<vi>, "Configuration Ref"=w490:refnum<vi>, "Action UI.Start Ref"=w489:refnum<vi>, "Action UI.Settings Ref"=w488:refnum<vi>, "Action UI.Exit Ref"=w487:refnum<vi>, "Action UI.Calibration Ref"=w486:refnum<vi>, "Action UI.Load Ref"=w485:refnum<vi>, "Action UI.Reset Ref"=w476:refnum<vi>)
        n184 = Build Array(w491, w490, w489, w488, w487, w486, w485, w476) -> (w479:refnum<vi>[])
        n185 = call "Set Enable State on Multiple Controls.vi"("Enable?"=TRUE, "Controls"=w479) -> ()  [unwired: 10 in]
        n186 = Unbundle By Name(w477) -> ("Action UI.Simuler Ref"=w484:refnum<vi>, "Action UI.Stop Ref"=w483:refnum<vi>, "Action UI.Save Ref"=w482:refnum<vi>)
        n187 = Build Array(w484, w483, w482) -> (w480:refnum<vi>[])
        n188 = call "Set Enable State on Multiple Controls.vi"("Enable?"=FALSE, "Controls"=w480) -> ()  [unwired: 10 in]
        n189 = Merge Errors(w495) -> (w494:errorcluster)
      }
      frame "Set UI Open Session" {
        # "Duplicate this frame when creating new messages.  Change this comment in the duplicated frame to describe this message."
        n190 = Unbundle By Name(w498) -> ("Status Ref"=w511:refnum<vi>, "Configuration Ref"=w510:refnum<vi>, "Action UI.Start Ref"=w509:refnum<vi>, "Action UI.Settings Ref"=w508:refnum<vi>, "Action UI.Exit Ref"=w507:refnum<vi>, "Action UI.Simuler Ref"=w506:refnum<vi>, "Action UI.Load Ref"=w505:refnum<vi>, "Action UI.Save Ref"=w497:refnum<vi>, "Action UI.Reset Ref"=w496:refnum<vi>)
        n191 = Build Array(w511, w510, w509, w508, w507, w506, w505, w497, w496) -> (w500:refnum<vi>[])
        n192 = call "Set Enable State on Multiple Controls.vi"("Enable?"=TRUE, "Controls"=w500) -> ()  [unwired: 10 in]
        n193 = Unbundle By Name(w498) -> ("Action UI.Calibration Ref"=w504:refnum<vi>, "Action UI.Stop Ref"=w503:refnum<vi>)
        n194 = Build Array(w504, w503) -> (w501:refnum<vi>[])
        n195 = call "Set Enable State on Multiple Controls.vi"("Enable?"=FALSE, "Controls"=w501) -> ()  [unwired: 10 in]
        n196 = Merge Errors(w515) -> (w514:errorcluster)
      }
      frame "Set UI Running" {
        # "Duplicate this frame when creating new messages.  Change this comment in the duplicated frame to describe this message."
        n197 = Unbundle By Name(w521) -> ("Status Ref"=w531:refnum<vi>, "Configuration Ref"=w530:refnum<vi>, "Action UI.Start Ref"=w529:refnum<vi>, "Action UI.Settings Ref"=w528:refnum<vi>, "Action UI.Exit Ref"=w527:refnum<vi>, "Action UI.Simuler Ref"=w526:refnum<vi>, "Action UI.Load Ref"=w525:refnum<vi>, "Action UI.Save Ref"=w520:refnum<vi>, "Action UI.Reset Ref"=w517:refnum<vi>, "Action UI.Calibration Ref"=w516:refnum<vi>)
        n198 = Build Array(w531, w530, w529, w528, w527, w526, w525, w520, w517, w516) -> (w522:refnum<vi>[])
        n199 = call "Set Enable State on Multiple Controls.vi"("Enable?"=FALSE, "Controls"=w522) -> ()  [unwired: 10 in]
        n200 = Unbundle By Name(w521) -> ("Action UI.Stop Ref"=w524:refnum<vi>)
        n201 = Build Array(w524) -> (w523:refnum<vi>[])
        n202 = call "Set Enable State on Multiple Controls.vi"("Enable?"=TRUE, "Controls"=w523) -> ()  [unwired: 10 in]
        n203 = Merge Errors(w535) -> (w534:errorcluster)
      }
      frame Default {
        # "'Default' case only runs if there is a message that isn't defined in any of the other cases.  Output a programming error."
        n204 = xnode "Error Ring"("parameter 0"=w537) -> ("error out"=w538:errorcluster)
      }
    }
    n205 = call "Error Handler - Message Handling Loop.vi"("error in (no error)"=w47, "Message Queue"=w45) -> ("dup error in"=w46:errorcluster)  [unwired: 8 in, 1 out]
  }
  n206 = while {
    tunnel: w17 -> [w553]
    tunnel: [w548] -> w40
    shift-right: [w552] -> w31
    shift-left: w38 -> [w554]
    stop <- w551 stop-if-true
    # "Event Handling Loop"
    n207 = event shown="[6] \"Calibrer\": Value Change" {
      selector: w554 -> [_ _ _ _ _ _ _ _ _ _ _ _]
      dyn-events: [_ _ _ _ _ _ _ _ _ _ _ _] -> w552
      timeout: _ -> [_ _ _ _ _ _ _ _ _ _ _ _]
      tunnel: [_ _ _ _ _ _ _ _ _ _ _ TRUE ("Discard?")] -> w551
      tunnel: w553 -> [w556 w561 w568 w572 w576 w579 w584 w585 w587 _ w591 w595]
      tunnel: [w558 w560 w563 w570 w575 w580 w582 _ w589 _ w594 _] -> w549
      tunnel: [w555 w559 w564 w571 w574 w578 w583 w585 w586 _ w590 w595] -> w550
      event "Start": Value Change {
        n208 = event-data() -> ()  [unwired: 1 in, 1 out]
        n209 = call-poly "Enqueue Message.vi"("Message"="Start", "Message Queue"=w556) -> ("error out"=w558:errorcluster, "dup Message Queue"=w555:refnum<queue>)  [unwired: 8 in]
      }
      event "Stop": Value Change {
        n210 = event-data() -> ()  [unwired: 1 in, 1 out]
        n211 = call-poly "Enqueue Message.vi"("Message"="Stop", "Message Queue"=w561) -> ("error out"=w560:errorcluster, "dup Message Queue"=w559:refnum<queue>)  [unwired: 8 in]
      }
      event Panel Close? {
        # "Send the 'Confirm Quit' message if the user closes the panel of the VI. Discard the event so the 'Confirm Quit' message has a chance to run."
        n212 = event-data() -> ()  [unwired: 1 in, 1 out]
        n213 = call-poly "Enqueue Message.vi"("Priority Message? (F)"=TRUE, "Message"="Confirm Quit", "Message Queue"=w568) -> ("error out"=w563:errorcluster, "dup Message Queue"=w564:refnum<queue>)  [unwired: 7 in]
        n214 = event-data("Discard?"=TRUE) -> ()  [unwired: 1 in, 1 out]
      }
      event "Enregistrer session": Value Change {
        n215 = event-data() -> ()  [unwired: 1 in, 1 out]
        n216 = call-poly "Enqueue Message.vi"("Message"="Save", "Message Queue"=w572) -> ("error out"=w570:errorcluster, "dup Message Queue"=w571:refnum<queue>)  [unwired: 8 in]
      }
      event "Charger session": Value Change {
        n217 = event-data() -> ()  [unwired: 1 in, 1 out]
        n218 = call-poly "Enqueue Message.vi"("Message"="Load", "Message Queue"=w576) -> ("error out"=w575:errorcluster, "dup Message Queue"=w574:refnum<queue>)  [unwired: 8 in]
      }
      event "Réinitialiser": Value Change {
        n219 = event-data() -> ()  [unwired: 1 in, 1 out]
        n220 = call-poly "Enqueue Message.vi"("Message"="Reset", "Message Queue"=w579) -> ("error out"=w580:errorcluster, "dup Message Queue"=w578:refnum<queue>)  [unwired: 8 in]
      }
      event "Calibrer": Value Change {
        n221 = event-data() -> ()  [unwired: 1 in, 1 out]
        n222 = call-poly "Enqueue Message.vi"("Message"="Calibrate", "Message Queue"=w584) -> ("error out"=w582:errorcluster, "dup Message Queue"=w583:refnum<queue>)  [unwired: 8 in]
      }
      event Application Instance Close {
        n223 = event-data() -> ()  [unwired: 1 in, 1 out]
      }
      event "Configuration.Avancée": Value Change {
        n224 = event-data() -> ()  [unwired: 1 in, 1 out]
        n225 = call-poly "Enqueue Message.vi"("Message"="Launch Settings Dialog", "Message Queue"=w587) -> ("error out"=w589:errorcluster, "dup Message Queue"=w586:refnum<queue>)  [unwired: 8 in]
      }
      event "Simuler": Value Change {
        n226 = event-data() -> ()  [unwired: 1 in, 1 out]
      }
      event "Exit": Value Change; Panel Close {
        w592 = TRUE  # Priority Message
        # "The UI Message Loop handles sending the Exit message to other loops."
        n227 = event-data() -> ()  [unwired: 1 in, 1 out]
        n228 = call-poly "Enqueue Message.vi"("Priority Message? (F)"=w592, "Message"="Exit", "Message Queue"=w591) -> ("error out"=w594:errorcluster, "dup Message Queue"=w590:refnum<queue>)  [unwired: 7 in]
      }
      event User Event {
        # "The Message Handling Loop processed an \"Exit\" message, which fired this event to stop the Event Handling Loop."
        n229 = event-data() -> ()  [unwired: 1 in, 1 out]
        n230 = local write "Status"("Exit" ("Exit String")) -> ()
      }
    }
    n231 = call "Error Handler - Event Handling Loop.vi"("error in (no error)"=w549, "Message Queue"=w550) -> ("dup error in"=w548:errorcluster)  [unwired: 8 in, 1 out]
  }
  n232 = call "Data Display.vi"("error in (no error)"=w19, "UI Data Display Cluster"=w4, "Message Queues in"=w16, "Notifier in"=w21) -> ("error out"=w18:errorcluster)  [unwired: 7 in]
  n233 = Unregister For Events(event registration refnum=w31, error in=w40) -> (error out=w32:errorcluster)
  n234 = Merge Errors(w32, w41, w36, w34, w26, w18) -> (w39:errorcluster)
  n235 = call "Destroy User Event - Stop.vi"("error in (no error)"=w39, "User Event - Stop"=w37) -> ("error out"=w27:errorcluster)  [unwired: 9 in]
  n236 = disable-structure shown="RUN_TIME_ENGINE==True" {
    disable-tunnel: w27 -> [_ _]
    frame condition #0 {
      # "Call Quit LabVIEW if running as a built application."
      n237 = Quit LabVIEW() -> ()  [unwired: 1 in]
    }
    frame condition #1 (active) {
    }
  }
